vi "Get Display Direction.vi"(8 "error in (no error)":errorcluster, 11 "senseHatDisplay in":refnum<class "RPI.SenseHat.Display.lvclass">) -> (0 "error out":errorcluster, 2 "Direction":T1, 3 "senseHatDisplay out":refnum<class "RPI.SenseHat.Display.lvclass">)   [LabVIEW 2020, in "RPI.SenseHat.Display.lvlib" / "RPI.SenseHat.Display.lvclass"]
doc: "Returns the direction of the screen."
uses:
  RPI.SenseHat.Display.lvclass
  TypeDefs/Display Direction.ctl
  RPI.SenseHat.Display.lvclass/RPI.SenseHat.Display.ctl
  RPI.SenseHat.Display.lvlib
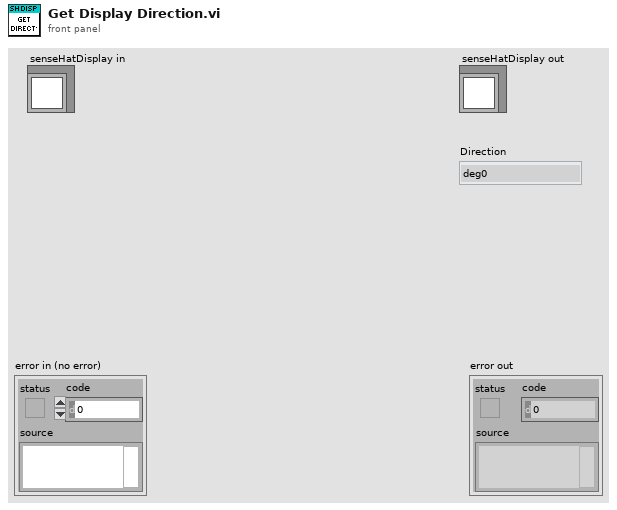
[diagram p1: front panel]
types:
  T1 = typedef "RPI.SenseHat.Display.lvlib/Display Direction.ctl" = enum16{"deg0", "deg90", "deg180", "deg270"}
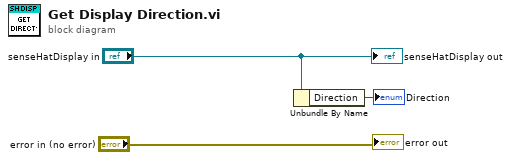
[diagram p0: block diagram]
diagram:
  n1 = Unbundle By Name("senseHatDisplay in") -> ("Direction"=→"Direction":T1)
  "error out" <- "error in (no error)"
  "senseHatDisplay out" <- "senseHatDisplay in"
